vi "validate default value.vi"(8 "error in":errorcluster, 11 "tag descriptor in":refnum<class "tag descriptor.lvclass">) -> (0 "error out":errorcluster, 2 "no default?":bool, 3 "tag descriptor out":refnum<class "tag descriptor.lvclass">)   [LabVIEW 2013, in "tag bus.lvlib" / "tag descriptor.lvclass"]
uses:
  tag descriptor.lvclass
  tag descriptor.lvclass/tag descriptor.ctl
  tag bus.lvlib
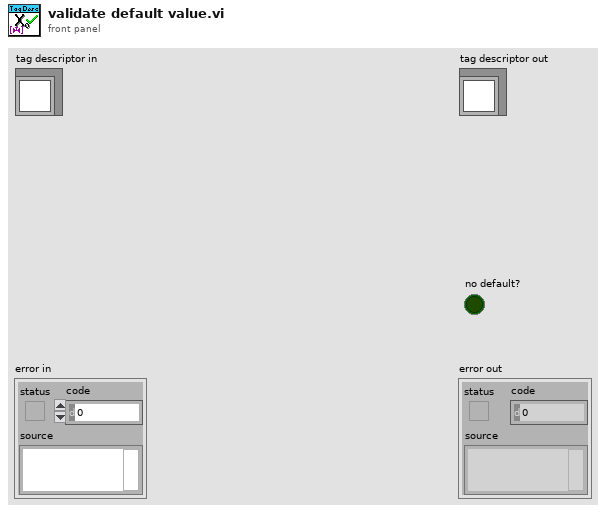
[diagram p1: front panel]
types:
  T1 = typedef "tag bus.lvlib/tag descriptor.lvclass/Data Type.ctl" = enum16{"Double", "Single", "I64", "I32", "I16", "I8", "U64", "U32", "U16", "U8", "Boolean", "String", "Array of Double", "Array of Single", "Array of I64", "Array of I32", "Array of I16", "Array of I8", "Array of U64", "Array of U32", "Array of U16", "Array of U8", "Array of Boolean", "Array of String"}
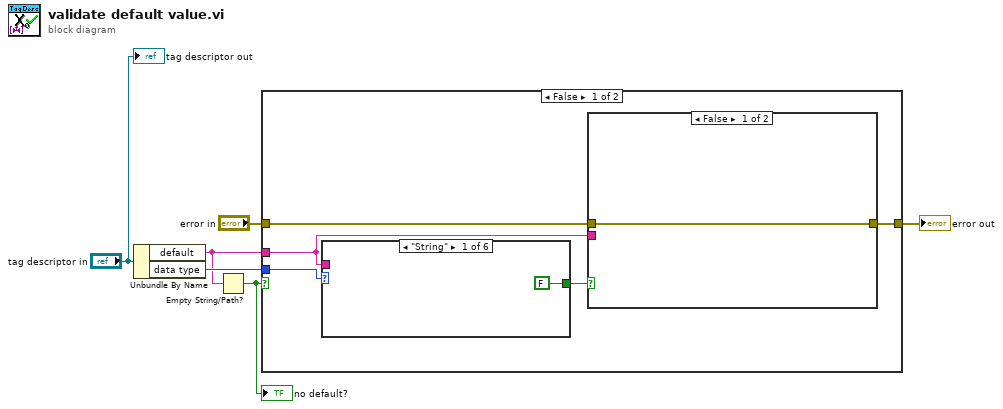
[diagram p0: block diagram]
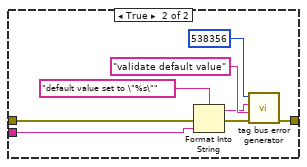
[diagram p2: hidden frame]
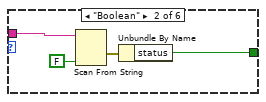
[diagram p3: hidden frame]
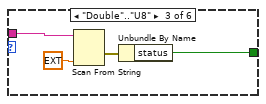
[diagram p4: hidden frame]
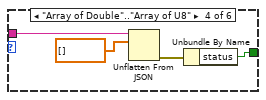
[diagram p5: hidden frame]
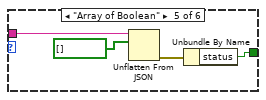
[diagram p6: hidden frame]
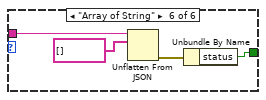
[diagram p7: hidden frame]
diagram:
  n1 = Unbundle By Name("tag descriptor in") -> ("default"=w1:string, "data type"=w2:T1)
  n2 = Empty String/Path?(string/path=w1) -> (empty?=w3:bool)
  "no default?" <- w3
  n3 = case shown="False" w3 {
    tunnel: [w9 w42] -> w5
    tunnel: "error in" -> [w8 w42]
    tunnel: w2 -> [w11 _]
    tunnel: w1 -> [w7 _]
    frame False {
      n4 = case shown="\"String\"" w11 {
        tunnel: [FALSE w23 w28 w31 w35 w39] -> w10
        tunnel: w7 -> [_ w22 w27 w30 w34 w38]
        frame "String" {
        }
        frame "Boolean" {
          n5 = Scan From String(input string=w22, default 1=FALSE) -> (error out=w24:errorcluster)  [unwired: 4 in, 2 out]
          n6 = Unbundle By Name(w24) -> ("status"=w23:bool)
        }
        frame "Double".."U8" {
          n7 = Scan From String(input string=w27, default 1=ext 0.0 ("default value 1")) -> (error out=w29:errorcluster)  [unwired: 4 in, 2 out]
          n8 = Unbundle By Name(w29) -> ("status"=w28:bool)
        }
        frame "Array of Double".."Array of U8" {
          n9 = Unflatten From JSON(JSON string=w30, type and defaults=dbl[] [] ("default value")) -> (error out=w32:errorcluster)  [unwired: 5 in, 1 out]
          n10 = Unbundle By Name(w32) -> ("status"=w31:bool)
        }
        frame "Array of Boolean" {
          n11 = Unflatten From JSON(JSON string=w34, type and defaults=bool[] [] ("default value")) -> (error out=w36:errorcluster)  [unwired: 5 in, 1 out]
          n12 = Unbundle By Name(w36) -> ("status"=w35:bool)
        }
        frame "Array of String" {
          n13 = Unflatten From JSON(JSON string=w38, type and defaults=string[] [] ("default value")) -> (error out=w40:errorcluster)  [unwired: 5 in, 1 out]
          n14 = Unbundle By Name(w40) -> ("status"=w39:bool)
        }
      }
      n15 = case shown="False" w10 {
        tunnel: [w12 w17] -> w9
        tunnel: w8 -> [w12 w19]
        tunnel: w7 -> [_ w13]
        frame False {
        }
        frame True {
          n16 = Format Into String(format string="default value set to \"%s\"" ("append error message"), error in=w19, w13) -> (resulting string=w15:string, error out=w18:errorcluster)  [unwired: 1 in]
          n17 = call "tag bus error generator.vi"("error in"=w18, "source"="validate default value", "append error message"=w15, "error code (0)"=538356) -> ("error out"=w17:errorcluster)  [unwired: 5 in]
        }
      }
    }
    frame True {
    }
  }
  "error out" <- w5
  "tag descriptor out" <- "tag descriptor in"
